vi "Do.vi"(8 "error in (no error)":errorcluster, 10 "Actor in":refnum<class "Actor.lvclass">, 11 "EMS Measurement Visualization Msg":refnum<class "EMS Measurement Visualization Msg.lvclass">) -> (0 "error out":errorcluster, 2 "Actor out":refnum<class "Actor.lvclass">)   [LabVIEW 2015, in "Master Controller Core.lvlib" / "EMS Measurement Visualization Msg.lvclass"]
doc: "This VI delivers the message to the actor by calling the appropriate method(s) on the actor."
uses:
  EMS Measurement Visualization Msg.lvclass
  <vilib>/ActorFramework/Actor/Actor.lvclass
  Master Controller/Master Controller.lvclass
  SCADA Core/SCADA Abstract Messages/IED Measurement Status Msg/IED Measurement Status Msg.lvclass/IED Measurement Status Msg.ctl
  SCADA Core/SCADA Abstract Messages/IED Measurement Status Msg/IED Measurement Status Msg.lvclass
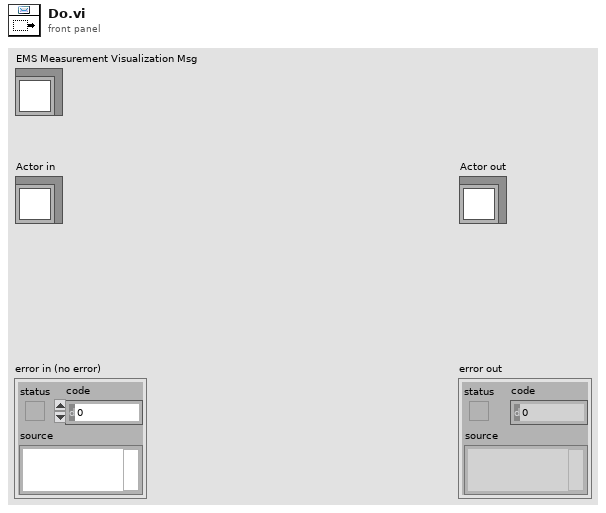
[diagram p1: front panel]
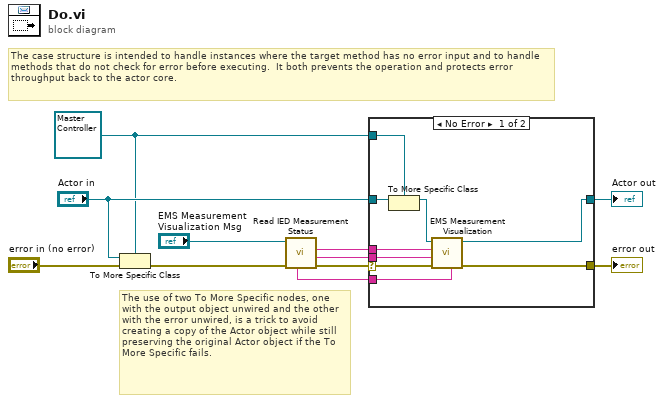
[diagram p0: block diagram]
diagram:
  w7 = refnum<class "Master Controller.lvclass"> refnum ("Actor in")
  # "The use of two To More Specific nodes, one with the output object unwired and the other with the error unwired, is a trick to avoid creating a copy of the Actor object while still preserving the original Actor object if the To More Specific fails."
  # "The case structure is intended to handle instances where the target method has no error input and to handle methods that do not check for error before executing.  It both prevents the operation and protects error throughput back to the actor core."
  n1 = To More Specific Class(target class=w7, reference="Actor in", error in="error in (no error)") -> (error out=w3:errorcluster)  [unwired: 1 out]
  n2 = call "Read IED Measurement Status.vi"("error in (no error)"=w3, "IED Measurement Msg in"="EMS Measurement Visualization Msg") -> ("error out"=w2:errorcluster, "Measurement Name"=w4:string, "IED Name"=w5:string, "Value/error"=w1:string)  [unwired: 4 in, 2 out]
  n3 = case shown="No Error" w2 {
    selector: w2 -> [w18 w22]
    tunnel: [w20 w22] -> w10
    tunnel: [w19 w21] -> w9
    tunnel: "Actor in" -> [w17 w21]
    tunnel: w7 -> [w16 _]
    tunnel: w5 -> [w14 _]
    tunnel: w4 -> [w13 _]
    tunnel: w1 -> [w12 _]
    frame No Error {
      n4 = To More Specific Class(target class=w16, reference=w17) -> (specific class reference=w15:refnum<class "Master Controller.lvclass">)  [unwired: 1 in, 1 out]
      n5 = call-dynamic "EMS Measurement Visualization.vi"("Measurement/Error"=w12, "error in (no error)"=w18, "Measurement Name"=w13, "IED Name"=w14, "Master Controller in"=w15) -> ("error out"=w20:errorcluster, "Master Controller out"=w19:refnum<class "Master Controller.lvclass">)  [unwired: 5 in]
    }
    frame Error {
      # "If type check fails, pass the original object out again."
    }
  }
  "error out" <- w10
  "Actor out" <- w9
